vi "Config.vi"(8 "error in (no error)":errorcluster, 11 "CAP-USB-1 in":refnum<class "CAP-USB-1.lvclass">) -> (0 "error out":errorcluster, 2 "Hal Config Data":T1, 3 "CAP-USB-1 out":refnum<class "CAP-USB-1.lvclass">)   [LabVIEW 2014, in "CAP-USB-1.lvlib" / "CAP-USB-1.lvclass"]
doc: "VI encargado de los parametros de configuracion del dispositivo"
uses:
  CAP-USB-1.lvclass
  DriverMasterSync/build/DriverMasterSync.lvlibp/Modules/HAL/TypeDefs/HAL Config Data.ctl
  DriverMasterSync/build/DriverMasterSync.lvlibp
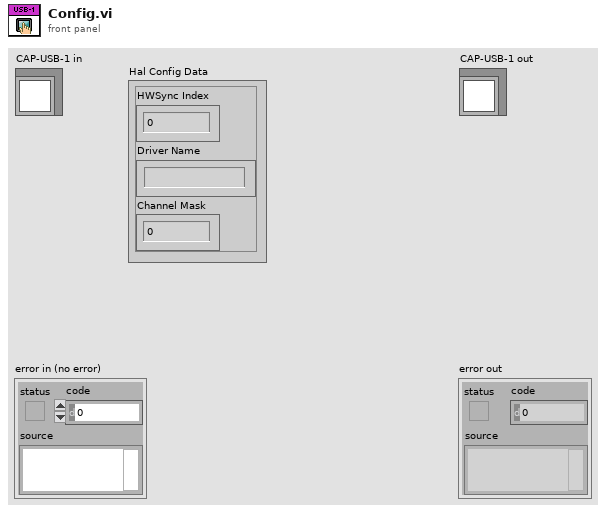
[diagram p1: front panel]
types:
  T1 = typedef "DriverMasterSync.lvlibp/HAL Config Data.ctl" = cluster{"HWSync Index":u32, "Driver Name":string, "Channel Mask":u64}
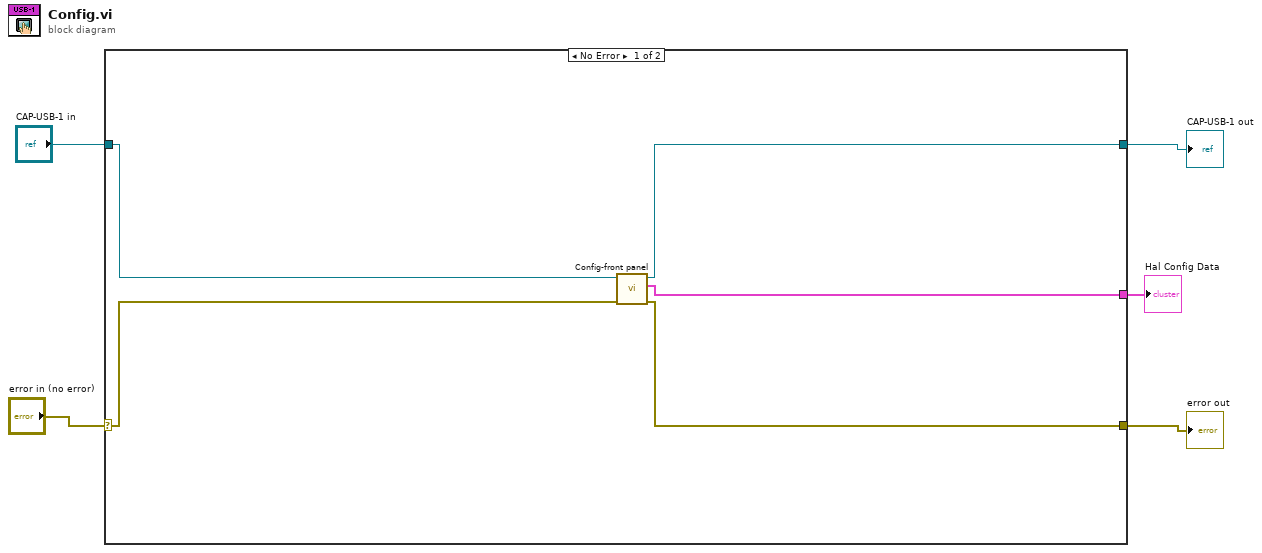
[diagram p0: block diagram]
diagram:
  n1 = case shown="No Error" "error in (no error)" {
    selector: "error in (no error)" -> [w9 w12]
    tunnel: [w7 w12] -> w4
    tunnel: [w8 w11] -> w2
    tunnel: "CAP-USB-1 in" -> [w10 w11]
    tunnel: [w6 _] -> w1
    frame No Error {
      n2 = call "Config-front panel.vi"("error in (no error)"=w9, "CAP-USB-1 in"=w10) -> ("error out"=w7:errorcluster, "output cluster"=w6:T1, "CAP-USB-1 out"=w8:refnum<class "CAP-USB-1.lvclass">)  [unwired: 7 in]
    }
    frame Error {
    }
  }
  "error out" <- w4
  "CAP-USB-1 out" <- w2
  "Hal Config Data" <- w1
